vi "Check Paddle Collision.vi"(6 "Screen Width":i16, 7 "Plot Width":u32, 9 "Paddle Radius":dbl, 10 "CursorX":i32, 11 "Ball X Position":dbl) -> (3 "Ball On Paddle?":bool)   [LabVIEW 2015]
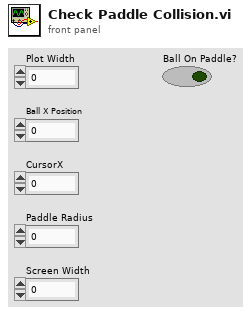
[diagram p1: front panel]
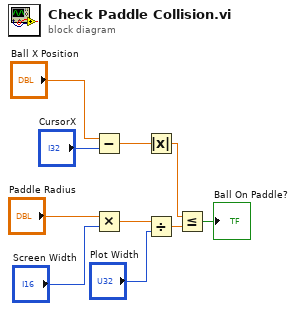
[diagram p0: block diagram]
diagram:
  n1 = Subtract(x="Ball X Position", y="CursorX") -> (x-y=w1:dbl)
  n2 = Multiply(x="Paddle Radius", y="Screen Width") -> (x*y=w5:dbl)
  n3 = Absolute Value(x=w1) -> (abs(x)=w2:dbl)
  n4 = Divide(x=w5, y="Plot Width") -> (x/y=w7:dbl)
  n5 = Less Or Equal?(x=w2, y=w7) -> (x <= y?=→"Ball On Paddle?":bool)
